vi "dcopy.vi"(4 "incy":i32, 6 "incx":i32, 7 "n":i32, 10 "dy":dbl[](array[numeric]), 11 "dx":dbl[](array[numeric])) -> (3 "dy_copied":dbl[](array[numeric]))   [LabVIEW 2014]
panel:
  out "mp1":i32
  out "m":i32=1
  out "iy":i32=1
  out "ix":i32=1
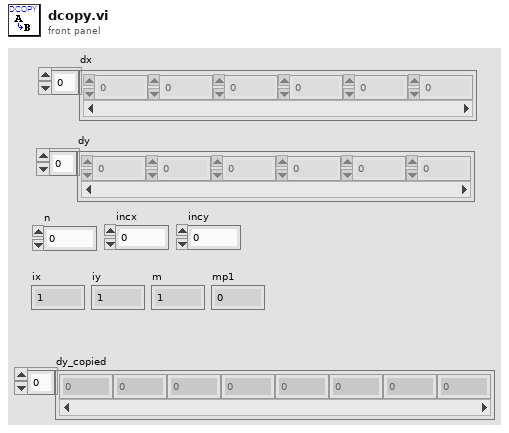
[diagram p1: front panel]
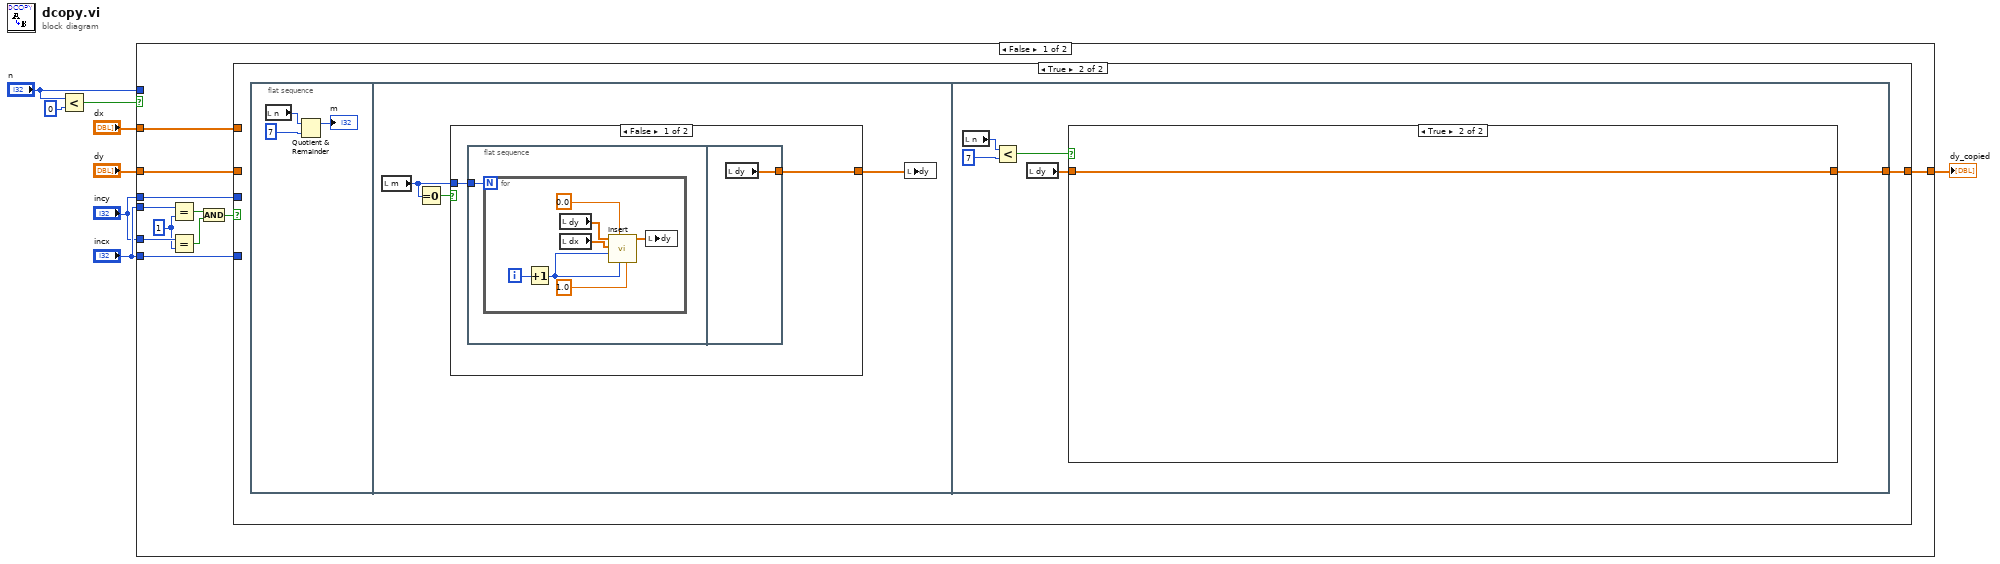
[diagram p0: block diagram]
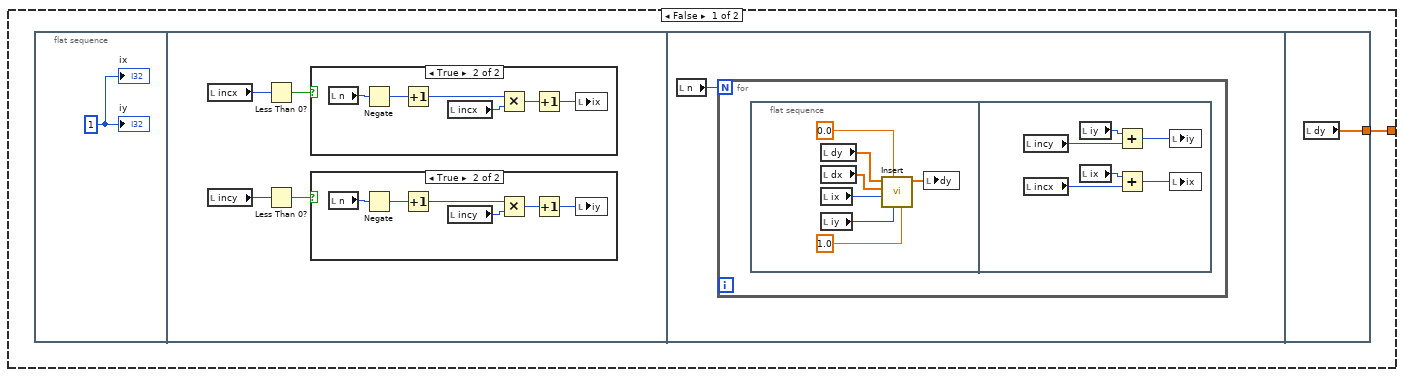
[diagram p2: hidden frame]
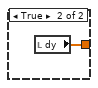
[diagram p5: hidden frame]
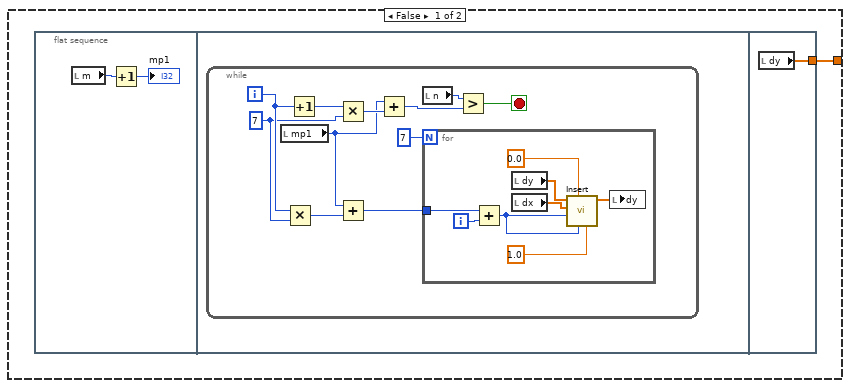
[diagram p6: hidden frame]
diagram:
  n1 = Less?(x="n", y=0) -> (x < y?=w8:bool)
  n2 = case shown="False" w8 {
    tunnel: "dy" -> [w14 w101]
    tunnel: [w9 w101] -> w1
    tunnel: "incx" -> [w19 _]
    tunnel: "dx" -> [w15 _]
    tunnel: "incy" -> [w18 _]
    tunnel: "n" -> [_ _]
    tunnel: "incx" -> [w17 _]
    tunnel: "incy" -> [w16 _]
    frame False {
      w13 = 1
      n3 = Equal?(x=w19, y=w13) -> (x = y?=w12:bool)
      n4 = Equal?(x=w18, y=w13) -> (x = y?=w11:bool)
      n5 = And(x=w12, y=w11) -> (x .and. y?=w10:bool)
      n6 = case shown="True" w10 {
        tunnel: w17 -> [_ _]
        tunnel: w16 -> [_ _]
        tunnel: w15 -> [_ _]
        tunnel: w14 -> [_ _]
        tunnel: [w20 w53] -> w9
        frame False {
          n7 = flat-sequence {
            tunnel: [w52] -> w20
            frame #0 {
              w21 = 1
              "ix" <- w21
              "iy" <- w21
            }
            frame #1 {
              n8 = local read "incx"() -> (w25:i32)
              n9 = local read "incy"() -> (w22:i32)
              n10 = Less Than 0?(x=w25) -> (x < 0?=w24:bool)
              n11 = Less Than 0?(x=w22) -> (x < 0?=w23:bool)
              n12 = case shown="True" w24 {
                frame False {
                }
                frame True {
                  n13 = local read "n"() -> (w37:i32)
                  n14 = Negate(x=w37) -> (-x=w36:i32)
                  n15 = Increment(x=w36) -> (x+1=w35:i32)
                  n16 = local read "incx"() -> (w34:i32)
                  n17 = Multiply(x=w35, y=w34) -> (x*y=w33:i32)
                  n18 = Increment(x=w33) -> (x+1=w32:i32)
                  n19 = local write "ix"(w32) -> ()
                }
              }
              n20 = case shown="True" w23 {
                frame False {
                }
                frame True {
                  n21 = local read "n"() -> (w31:i32)
                  n22 = Negate(x=w31) -> (-x=w30:i32)
                  n23 = Increment(x=w30) -> (x+1=w29:i32)
                  n24 = local read "incy"() -> (w28:i32)
                  n25 = Multiply(x=w29, y=w28) -> (x*y=w27:i32)
                  n26 = Increment(x=w27) -> (x+1=w26:i32)
                  n27 = local write "iy"(w26) -> ()
                }
              }
            }
            frame #2 {
              n28 = local read "n"() -> (w38:i32)
              n29 = for {
                N: w38 -> [_]
                n30 = flat-sequence {
                  frame #0 {
                    n31 = local read "dy"() -> (w43:dbl[])
                    n32 = local read "dx"() -> (w42:dbl[])
                    n33 = local read "ix"() -> (w45:i32)
                    n34 = local read "iy"() -> (w44:i32)
                    n35 = call "Insert.vi"("da"=1.0 ("dy weight"), "iy"=w44, "dy weight"=0.0, "ix"=w45, "dx"=w42, "dy in"=w43) -> ("dy out"=w41:dbl[])  [unwired: 5 in]
                    n36 = local write "dy"(w41) -> ()
                  }
                  frame #1 {
                    n37 = local read "incy"() -> (w47:i32)
                    n38 = local read "incx"() -> (w50:i32)
                    n39 = local read "iy"() -> (w46:i32)
                    n40 = local read "ix"() -> (w51:i32)
                    n41 = Add(x=w46, y=w47) -> (x+y=w48:i32)
                    n42 = Add(x=w51, y=w50) -> (x+y=w49:i32)
                    n43 = local write "iy"(w48) -> ()
                    n44 = local write "ix"(w49) -> ()
                  }
                }
              }
            }
            frame #3 {
              n45 = local read "dy"() -> (w52:dbl[])
            }
          }
        }
        frame True {
          n46 = flat-sequence {
            tunnel: [w72] -> w53
            frame #0 {
              n47 = local read "n"() -> (w55:i32)
              n48 = Quotient & Remainder(x=w55, y=7) -> (x-y*floor(x/y)=→"m":i32)  [unwired: 1 out]
            }
            frame #1 {
              n49 = local read "m"() -> (w58:i32)
              n50 = Equal To 0?(x=w58) -> (x = 0?=w59:bool)
              n51 = case shown="False" w59 {
                tunnel: [w60 w71] -> w57
                tunnel: w58 -> [w61 _]
                frame False {
                  n52 = flat-sequence {
                    tunnel: w61 -> [w62]
                    tunnel: [w70] -> w60
                    frame #0 {
                      n53 = for {
                        N: w62 -> [_]
                        i -> [w69]
                        n54 = Increment(x=w69) -> (x+1=w68:i32)
                        n55 = local read "dy"() -> (w66:dbl[])
                        n56 = local read "dx"() -> (w67:dbl[])
                        n57 = call "Insert.vi"("da"=1.0, "iy"=w68, "dy weight"=0.0, "ix"=w68, "dx"=w67, "dy in"=w66) -> ("dy out"=w65:dbl[])  [unwired: 5 in]
                        n58 = local write "dy"(w65) -> ()
                      }
                    }
                    frame #1 {
                      n59 = local read "dy"() -> (w70:dbl[])
                    }
                  }
                }
                frame True {
                  n60 = local read "dy"() -> (w71:dbl[])
                }
              }
              n61 = local write "dy"(w57) -> ()
            }
            frame #2 {
              n62 = local read "n"() -> (w75:i32)
              n63 = Less?(x=w75, y=7) -> (x < y?=w74:bool)
              n64 = local read "dy"() -> (w76:dbl[])
              n65 = case shown="True" w74 {
                tunnel: w76 -> [_ w100]
                tunnel: [w77 w100] -> w72
                frame False {
                  n66 = flat-sequence {
                    tunnel: [w99] -> w77
                    frame #0 {
                      n67 = local read "m"() -> (w79:i32)
                      n68 = Increment(x=w79) -> (x+1=→"mp1":i32)
                    }
                    frame #1 {
                      n69 = while {
                        i -> [w83]
                        stop <- w86 stop-if-true
                        w82 = 7
                        n70 = local read "mp1"() -> (w81:i32)
                        n71 = Multiply(x=w83, y=w82) -> (x*y=w84:i32)
                        n72 = Increment(x=w83) -> (x+1=w90:i32)
                        n73 = Multiply(x=w90, y=w82) -> (x*y=w89:i32)
                        n74 = Add(x=w81, y=w84) -> (x+y=w80:i32)
                        n75 = Add(x=w81, y=w89) -> (x+y=w88:i32)
                        n76 = local read "n"() -> (w87:i32)
                        n77 = for {
                          N: 7 -> [_]
                          tunnel: w80 -> [w98]
                          i -> [w97]
                          n78 = Add(x=w98, y=w97) -> (x+y=w96:i32)
                          n79 = local read "dy"() -> (w94:dbl[])
                          n80 = local read "dx"() -> (w93:dbl[])
                          n81 = call "Insert.vi"("da"=1.0, "iy"=w96, "dy weight"=0.0, "ix"=w96, "dx"=w93, "dy in"=w94) -> ("dy out"=w95:dbl[])  [unwired: 5 in]
                          n82 = local write "dy"(w95) -> ()
                        }
                        n83 = Greater?(x=w87, y=w88) -> (0:w86:bool)
                      }
                    }
                    frame #2 {
                      n84 = local read "dy"() -> (w99:dbl[])
                    }
                  }
                }
                frame True {
                }
              }
            }
          }
        }
      }
    }
    frame True {
    }
  }
  "dy_copied" <- w1
